vi "Save Rename VI.vi"(8 "error in":errorcluster, 9 "Rename":string, 10 "VI Ref":refnum<vi>) -> (0 "error out":errorcluster)   [LabVIEW 2021, in "_Rename.lvlib" / "_Rename.lvclass"]
uses:
  _Rename.lvclass
  _Rename.lvclass/_Rename.ctl
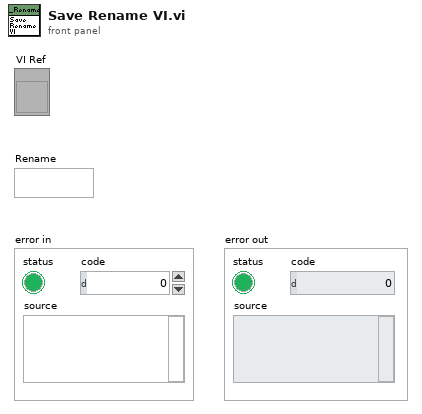
[diagram p1: front panel]
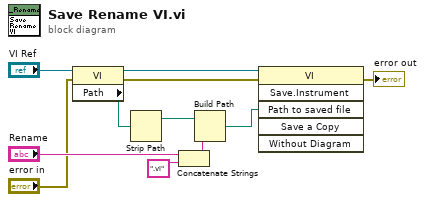
[diagram p0: block diagram]
diagram:
  n1 = property class="VI"(reference="VI Ref", error in="error in") -> (reference out=w5:refnum<vi>, error out=w6:errorcluster, "Path"=w8:path)
  n2 = Strip Path(path=w8) -> (stripped path=w10:path)  [unwired: 1 out]
  n3 = Concatenate Strings("Rename", ".vi" ("string")) -> (w7:string)
  n4 = Build Path(base path=w10, name or relative path=w7) -> (appended path=w11:path)
  n5 = invoke class="VI" method="Save.Instrument"(reference=w5, error in=w6, "Path to saved file"=w11) -> (error out=→"error out":errorcluster)  [unwired: 3 in, 5 out]
